vi "udp_validation.vi"() -> ()   [LabVIEW 2014]
panel:
  in  "ROS UDP Validation Value":u16 format="%x"
  # "This is used to verify the authenticity of a received \nUDP packet. If the first item transmitted in the string\nis not this value, the packet will be discarded."
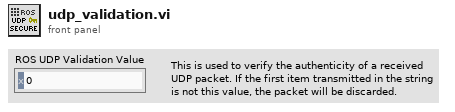
[diagram p1: front panel]
diagram:
